vi "Write To Spreadsheet File wheaders.vi"(0 "delimiter (\\t)":string="\t", 1 "transpose? (no:F)":bool, 2 "Headers":string[](array[string]), 4 "format (%s)":string="%s", 5 "append to file? (new file:F)":bool, 6 "1D data":string[](array[string]), 7 "2D data":string[][](array[string]), 8 "file path (dialog if empty)":path) -> (3 "new file path (Not A Path if cancelled)":path)   [LabVIEW 2011]
doc: "Converts a 2D or 1D array of strings, signed integers, or double-precision numbers to a text string and writes the string to a new byte stream file or appends the string to an existing file. Wire data to the <B>2D data</B> input or <B>1D data</B> input to determine the polymorphic instance to use or manually select the instance.\n\nUse this VI to transpose or separate data.\n\n<B>Note</B> To format with Microsoft Excel, use ActiveX with LabVIEW or the Report Generation Toolkit for Microsoft Office."
uses:
  <vilib>/Utility/error.llb/DialogType.ctl
panel:
  in  "prompt":string="Choose file to write."
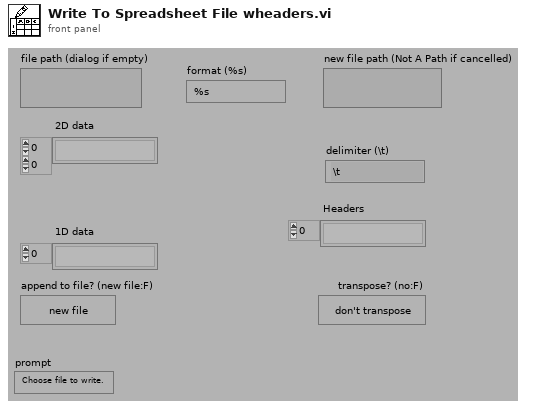
[diagram p1: front panel]
types:
  T1 = typedef "DialogType.ctl" = u16
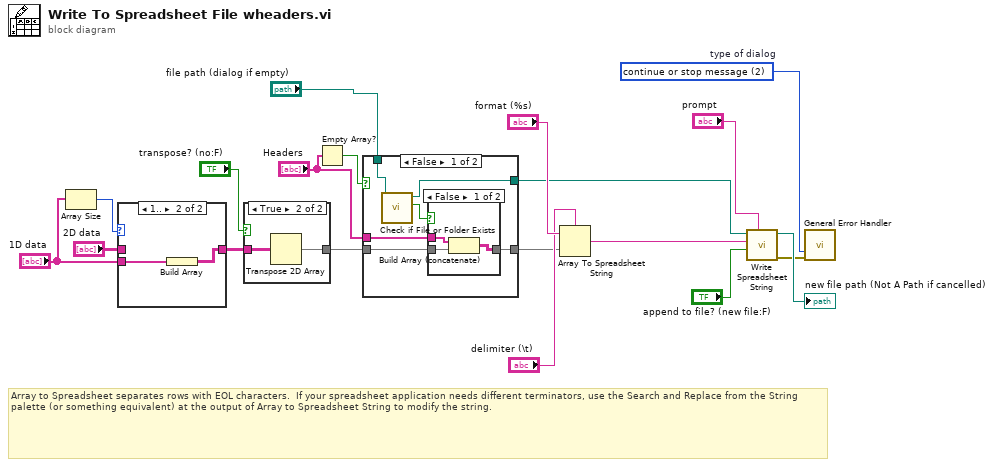
[diagram p0: block diagram]
diagram:
  w7 = T1 2 items=["no dialog", "OK message", "continue or stop message", "OK message + warnings", "continue/stop + warnings"]  # type of dialog
  # "Array to Spreadsheet separates rows with EOL characters.  If your spreadsheet application needs different terminators, use the Search and Replace from the String palette (or something equivalent) at the output of Array to Spreadsheet String to modify the string."
  n1 = Array Size(array="1D data") -> (size(s)=w19:i32)
  n2 = case shown="1.." w19 {
    tunnel: "1D data" -> [_ w22]
    tunnel: [w20 w21] -> w15
    tunnel: "2D data" -> [w20 _]
    frame ..0 {
      # "1D array is empty"
    }
    frame 1.. {
      n3 = Build Array(w22) -> (w21:string[][])
    }
  }
  n4 = case shown="True" "transpose? (no:F)" {
    tunnel: [w23 w25] -> w4
    tunnel: w15 -> [w23 w24]
    frame False {
    }
    frame True {
      n5 = Transpose 2D Array(2D array=w24) -> (transposed array=w25:string[][])
    }
  }
  n6 = Empty Array?(array="Headers") -> (empty?=w6:bool)
  n7 = case shown="False" w6 {
    tunnel: w4 -> [w31 w37]
    tunnel: "Headers" -> [w30 _]
    tunnel: [w29 w37] -> w3
    tunnel: "file path (dialog if empty)" -> [w28 w36]
    tunnel: [w26 w36] -> w1
    frame False {
      n8 = call <vilib>:"Check if File or Folder Exists.vi"("path"=w28) -> ("file or folder exists?"=w27:bool, "dup path"=w26:path)  [unwired: 8 in, 1 out]
      n9 = case shown="False" w27 {
        tunnel: w31 -> [w34 w35]
        tunnel: w30 -> [w33 _]
        tunnel: [w32 w35] -> w29
        frame False {
          n10 = Build Array (concatenate)(w33, w34) -> (w32:string[][])
        }
        frame True {
        }
      }
    }
    frame True {
    }
  }
  n11 = Array To Spreadsheet String(delimiter (Tab)="delimiter (\\t)", array=w3, 3:"format (%s)") -> (spreadsheet string=w9:string)
  n12 = call <vilib>:"Write Spreadsheet String.vi"("prompt"="prompt", "append to file? (new file:F)"="append to file? (new file:F)", "spreadsheet string"=w9, "file path (dialog if empty)"=w1) -> ("error out"=w8:errorcluster, "path"=→"new file path (Not A Path if cancelled)":path)  [unwired: 6 in]
  n13 = call <vilib>:"General Error Handler.vi"("type of dialog (OK msg:1)"=w7, "error in (no error)"=w8) -> ()  [unwired: 9 in, 5 out]
